vi "sync end of cycle.vi"(8 "error in (no error)":errorcluster, 10 "parameters data in":T1, 11 "module in":refnum<class "Shared Memory runtime.lvclass">) -> (0 "error out":errorcluster, 2 "parameters data out":T1, 3 "module out":refnum<class "Shared Memory runtime.lvclass">)   [LabVIEW 2014, in "Shared Memory runtime.lvclass"]
uses:
  Shared Memory runtime.lvclass
  <vilib>/NI/Tag Bus/table/data table.lvlib
  <vilib>/NI/Tag Bus/table/data polymorphs/read one/read Double.vi
  <vilib>/NI/Tag Bus/table/data table.ctl
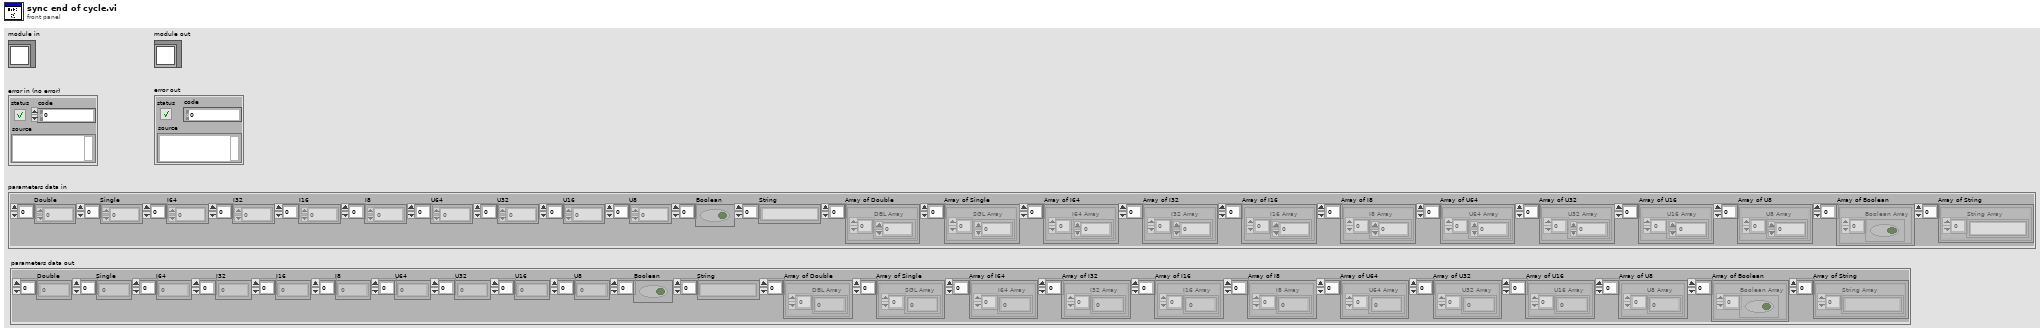
[diagram p1: front panel]
types:
  T1 = typedef "tag bus.lvlib/data table.lvlib/data table.ctl" = cluster{"Double":dbl[], "Single":sgl[], "I64":i64[], "I32":i32[], "I16":i16[], "I8":i8[], "U64":u64[], "U32":u32[], "U16":u16[], "U8":u8[], "Boolean":bool[], "String":string[], "Array of Double":cluster{"DBL Array":dbl[]}[], "Array of Single":cluster{"SGL Array":sgl[]}[], "Array of I64":cluster{"I64 Array":i64[]}[], "Array of I32":cluster{"I32 Array":i32[]}[], "Array of I16":cluster{"I16 Array":i16[]}[], "Array of I8":cluster{"I8 Array":i8[]}[], "Array of U64":cluster{"U64 Array":u64[]}[], "Array of U32":cluster{"U32 Array":u32[]}[], "Array of U16":cluster{"U16 Array":u16[]}[], "Array of U8":cluster{"U8 Array":u8[]}[], "Array of Boolean":cluster{"Boolean Array":bool[]}[], "Array of String":cluster{"String Array":string[]}[]}
  T2 = typedef "Shared Memory runtime.lvclass/sync data.ctl" = cluster{"semaphores soc":T3[], "semaphores eoc":T3[], "timeout":dbl, "enabled":bool, "sync shared memory":T5, "publish timing":bool, "timing indices":T6, "timing pointers":T7}
  T3 = typedef "Shared Memory runtime.lvclass/semaphore data.ctl" = cluster{"semaphore":T4, "name":string}
  T4 = typedef "POSIX Threads.lvlib/Semaphore.lvclass/reference.ctl" = refnum<data-value>
  T5 = typedef "Shared Memory.lvlib/Shared Memory.lvclass/reference.ctl" = refnum<data-value>
  T6 = typedef "Shared Memory runtime.lvclass/sync timing indices.ctl" = cluster{"start time index":i32}
  T7 = typedef "Shared Memory runtime.lvclass/sync timing pointers.ctl" = cluster{"start sec ptr":u64, "start nsec ptr":u64}
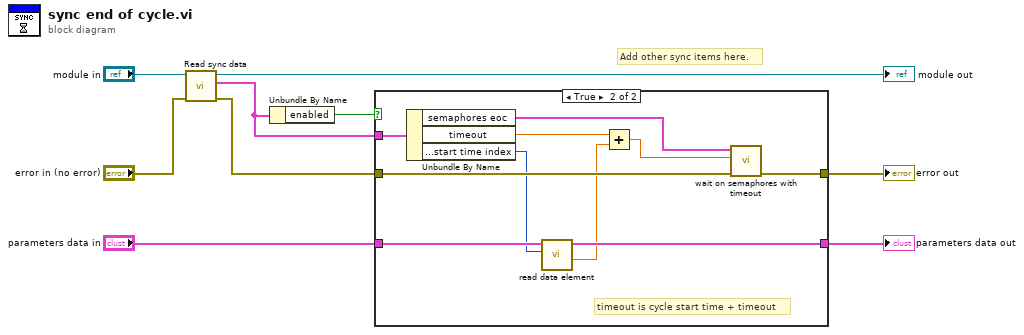
[diagram p0: block diagram]
diagram:
  # "Add other sync items here."
  n1 = call "Read sync data.vi"("error in (no error)"="error in (no error)", "Shared Memory runtime in"="module in") -> ("error out"=w2:errorcluster, "sync data"=w1:T2, "Shared Memory runtime out"=→"module out":refnum<class "Shared Memory runtime.lvclass">)  [unwired: 7 in]
  n2 = Unbundle By Name(w1) -> ("enabled"=w8:bool)
  n3 = case shown="True" w8 {
    tunnel: w2 -> [w11 w21]
    tunnel: [w11 w20] -> w9
    tunnel: "parameters data in" -> [w10 w19]
    tunnel: [w10 w18] -> w6
    tunnel: w1 -> [_ w17]
    frame False {
    }
    frame True {
      # "timeout is cycle start time + timeout"
      n4 = Unbundle By Name(w17) -> ("semaphores eoc"=w15:T3[], "timeout"=w14:dbl, "timing indices.start time index"=w16:i32)
      n5 = call-poly <vilib>:"read data element.vi"("index"=w16, "data table in"=w19) -> ("value"=w13:dbl, "data table out"=w18:T1)  [unwired: 8 in]
      n6 = Add(x=w14, y=w13) -> (x+y=w12:dbl)
      n7 = call "wait on semaphores with timeout.vi"("error in (no error)"=w21, "abs sec timeout"=w12, "semaphores in"=w15) -> ("error out"=w20:errorcluster)  [unwired: 7 in, 1 out]
    }
  }
  "error out" <- w9
  "parameters data out" <- w6
